vi "Linear Programming Preparation (I64).vi"(8 "dim2(M)":i32, 9 "dim1 (M)":i32, 10 "M":i64[][](array[numeric]), 11 "B":i64[](array[numeric])) -> (0 "dim1+dim2":i32, 1 "n-m":u32[](array[numeric]), 2 "m":u32[](array[numeric]), 3 "Table":i64[][](array[numeric]))   [LabVIEW 2025, in "AOC.lvlib"]
uses:
  AOC.lvlib
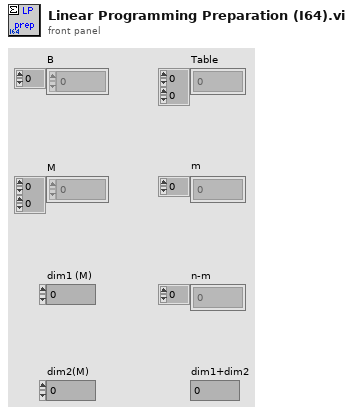
[diagram p1: front panel]
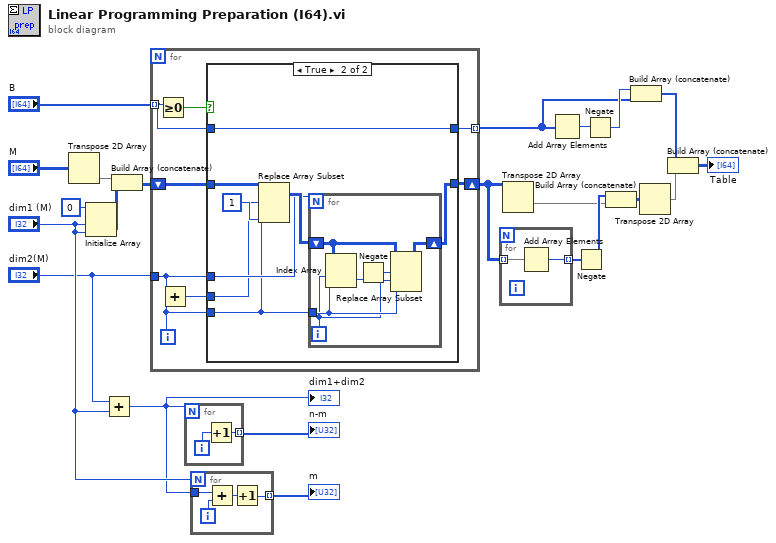
[diagram p0: block diagram]
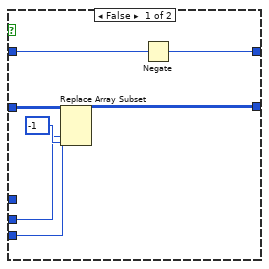
[diagram p2: hidden frame]
diagram:
  n1 = Transpose 2D Array(2D array="M") -> (transposed array=w19:i64[][])
  n2 = Initialize Array(i64 0, "dim1 (M)", "dim1 (M)") -> (w20:i64[][])
  n3 = Add(x="dim2(M)", y="dim1 (M)") -> (x+y=w1:i32)
  "dim1+dim2" <- w1
  n4 = Build Array (concatenate)(w19, w20) -> (w16:i64[][])
  n5 = for {
    tunnel: "B" -> [w24] mode=indexing
    tunnel: "dim2(M)" -> [w25]
    shift-right: [w26] -> w2
    shift-left: w16 -> [w27]
    tunnel: [w23] -> w12 mode=indexing
    i -> [w28]
    n6 = Greater Or Equal To 0?(x=w24) -> (x >= 0?=w30:bool)
    n7 = Add(x=w25, y=w28) -> (x+y=w29:i32)
    n8 = case shown="True" w30 {
      tunnel: w29 -> [w32 w40]
      tunnel: w28 -> [w33 w39]
      tunnel: w27 -> [w36 w44]
      tunnel: [w35 w42] -> w26
      tunnel: w25 -> [_ w41]
      tunnel: w24 -> [w34 w38]
      tunnel: [w31 w38] -> w23
      frame False {
        n9 = Replace Array Subset(array=w36, new element=i64 -1, index (row)=w32, index (col)=w33) -> (w35:i64[][])
        n10 = Negate(x=w34) -> (-x=w31:i64)
      }
      frame True {
        n11 = Replace Array Subset(array=w44, new element=i64 1, index (row)=w40, index (col)=w39) -> (w43:i64[][])
        n12 = for {
          N: w41 -> [_]
          shift-right: [w51] -> w42
          shift-left: w43 -> [w50]
          tunnel: w39 -> [w47]
          i -> [w46]
          n13 = Index Array(array=w50, index (row)=w46, index (col)=w47) -> (element=w49:i64)
          n14 = Negate(x=w49) -> (-x=w48:i64)
          n15 = Replace Array Subset(array=w50, new element=w48, index (row)=w46, index (col)=w47) -> (w51:i64[][])
        }
      }
    }
  }
  n16 = for {
    N: w1 -> [_]
    tunnel: [w52] -> w14 mode=indexing
    i -> [w53]
    n17 = Increment(x=w53) -> (x+1=w52:i32)
  }
  "n-m" <- w14
  n18 = for {
    N: "dim1 (M)" -> [_]
    tunnel: w1 -> [w57]
    tunnel: [w54] -> w3 mode=indexing
    i -> [w56]
    n19 = Add(x=w57, y=w56) -> (x+y=w55:i32)
    n20 = Increment(x=w55) -> (x+1=w54:i32)
  }
  "m" <- w3
  n21 = for {
    tunnel: w2 -> [w59] mode=indexing
    tunnel: [w58] -> w17 mode=indexing
    n22 = Add Array Elements(numeric array=w59) -> (sum=w58:i64)
  }
  n23 = Transpose 2D Array(2D array=w2) -> (transposed array=w8:i64[][])
  n24 = Add Array Elements(numeric array=w12) -> (sum=w15:i64)
  n25 = Negate(x=w17) -> (-x=w11:i64[])
  n26 = Negate(x=w15) -> (-x=w13:i64)
  n27 = Build Array (concatenate)(w11, w8) -> (w7:i64[][])
  n28 = Build Array (concatenate)(w13, w12) -> (w10:i64[])
  n29 = Transpose 2D Array(2D array=w7) -> (transposed array=w6:i64[][])
  n30 = Build Array (concatenate)(w10, w6) -> (→"Table":i64[][])
